vi "PolarizerRotator.vi"() -> ()   [LabVIEW 2022 SP3]
uses:
  Control_rotator.ctl
  <vilib>/Analysis/baseanly.llb/Mean (DBL).vi
  <vilib>/Analysis/NI_AALBase.lvlib
panel:
  out "error out":errorcluster
  out "concatenated string":string="0mr000007C6"
  out "Waveform Graph 2":dbl[](graph)=[0.0114104102289922, 0.005331864005048672, 0.002365437653122095, 0.0020399943555791337, 0.0018238947466399568, 0.0038770713125236265, 0.009183223773610314, 0.017346081821373458, 0.028008969359547123, 0.040766102580344826, 0.056787694052, 0.07599250286066472, 0.09984112907767431, 0.12767396257315167, 0.15908169019639953, 0.1934532823915446, 0.22536977633845853, 0.25900355543902787, 0.2854221431566561, 0.31011831747145174, 0.3226821647724511, 0.32980024781774636, 0.3281776128886943, 0.3166476606516057, 0.2977695101545653, 0.26886629570979925, 0.24020462092063113, 0.20869158381742006, 0.1768178373750466, 0.146450811441169, 0.11622057138066992, 0.09032385739868065, 0.06709021181202998, 0.04842705992607135, 0.03356983053430435, 0.021401558819280752, 0.012115542962350739]
  out "Waveform Graph":dbl[](graph)
  in  "Divide":bool
  in  "Store reference":bool
  out "String":string="000007C6"
  in  "Jog size (degrees)":dbl=5.0
  in  "Set jog size":bool
  in  "Cancel":bool
  in  "Sweep angle":dbl=180.0
  out "Current angle":i32=180
  in  "Home":bool
  in  "stop":bool
  in  "Jog":bool
  in  "milliseconds to wait":u32=1000
  out "read buffer":string="0POFFFFFFFD\r\n"
  in  "VISA resource name":refnum<visa-resource-name>="COM3"
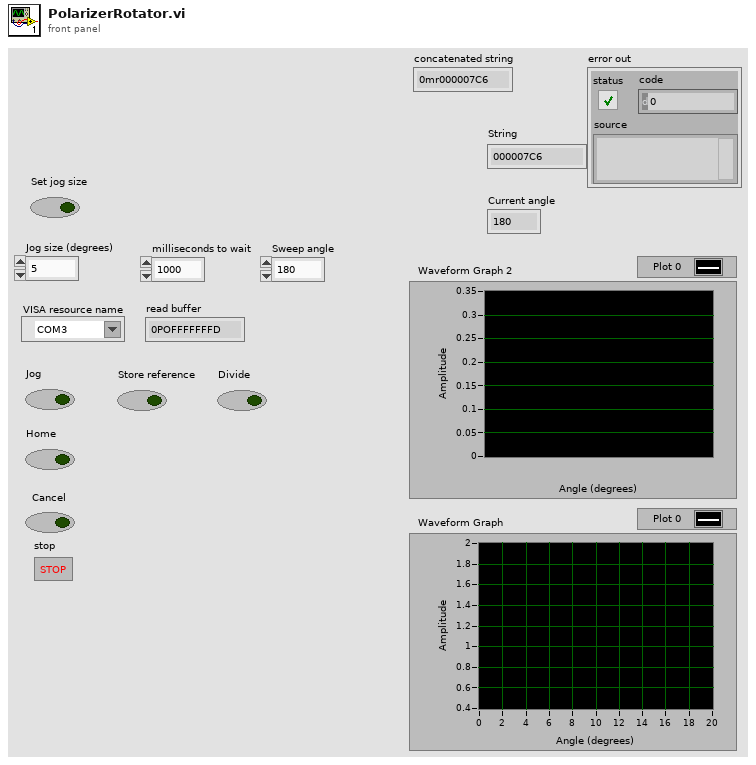
[diagram p1: front panel]
types:
  T1 = typedef "Control_rotator.ctl" = enum16{"Sit Idle", "Jog", "Set Jog Size", "Home", "Store reference", "Divide"}
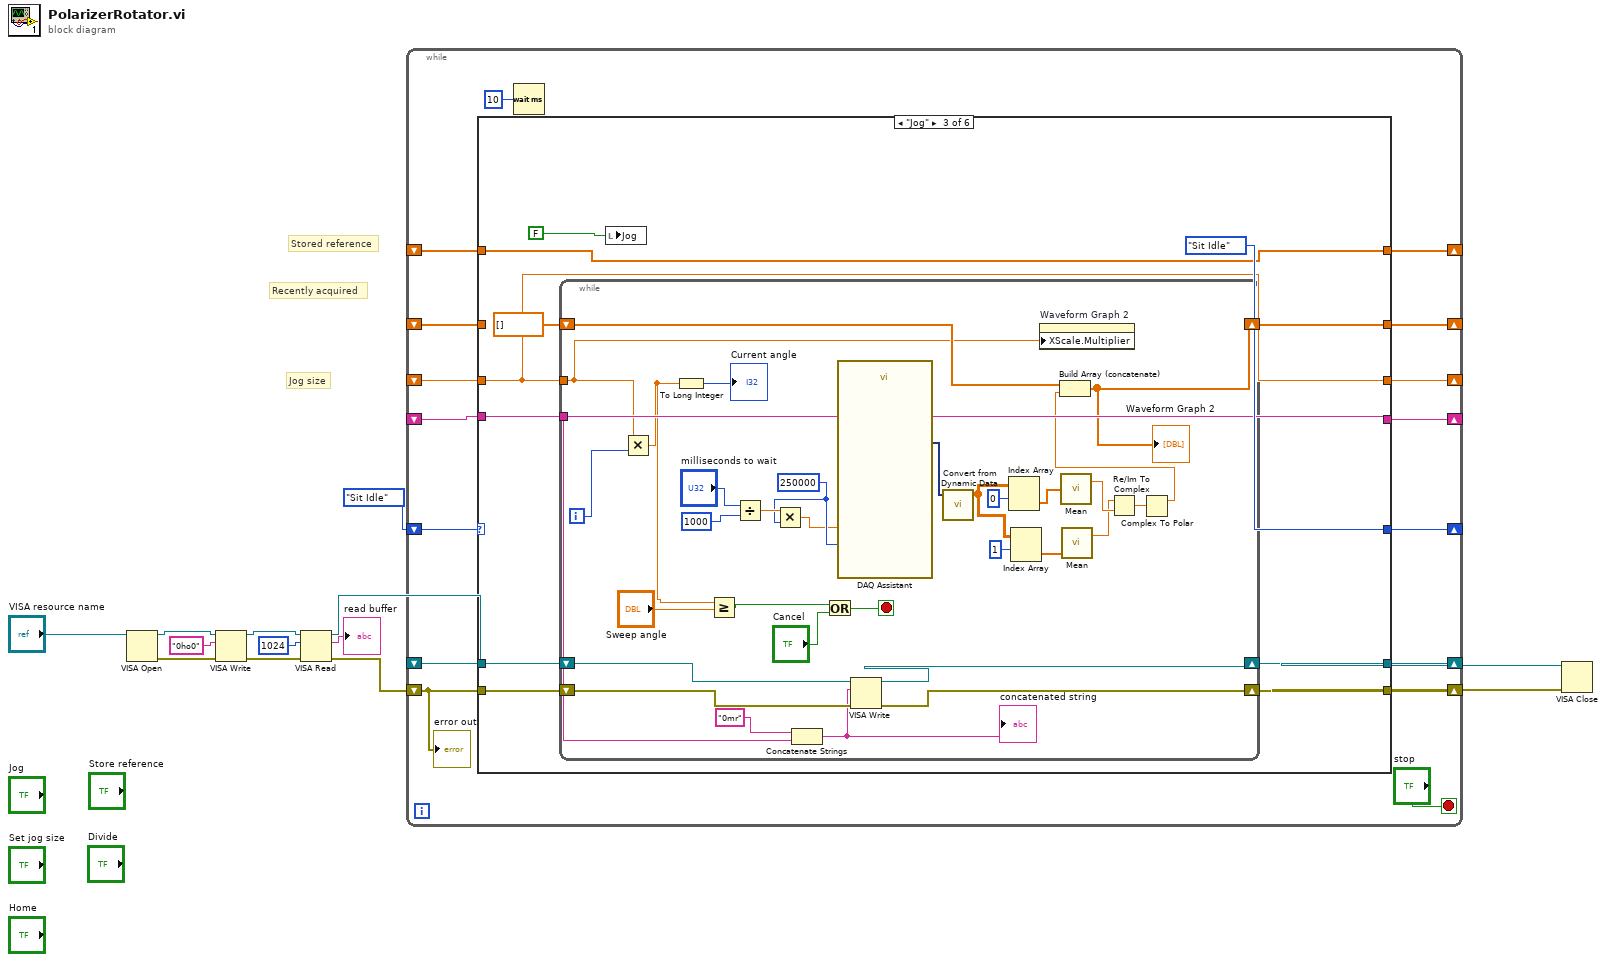
[diagram p0: block diagram]
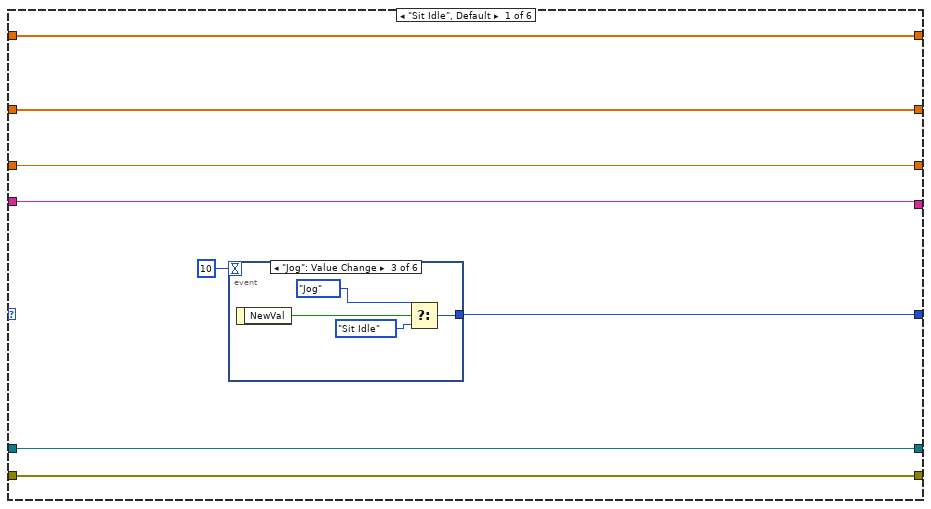
[diagram p2: hidden frame]
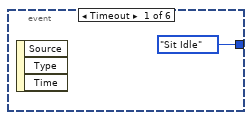
[diagram p3: hidden frame]
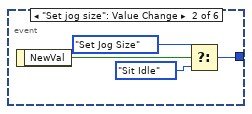
[diagram p4: hidden frame]
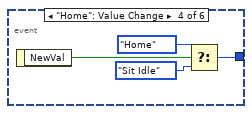
[diagram p5: hidden frame]
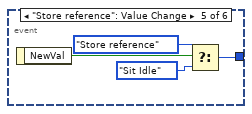
[diagram p6: hidden frame]
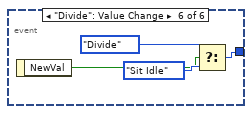
[diagram p7: hidden frame]
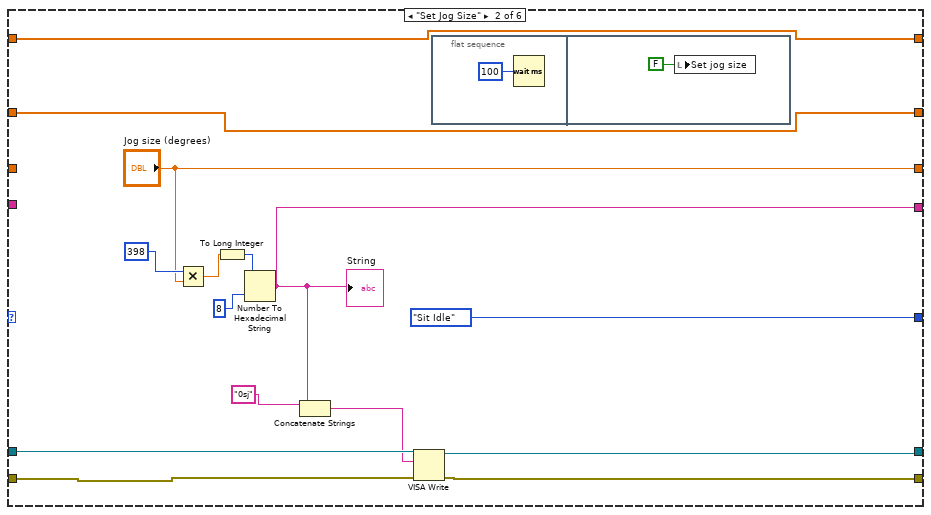
[diagram p8: hidden frame]
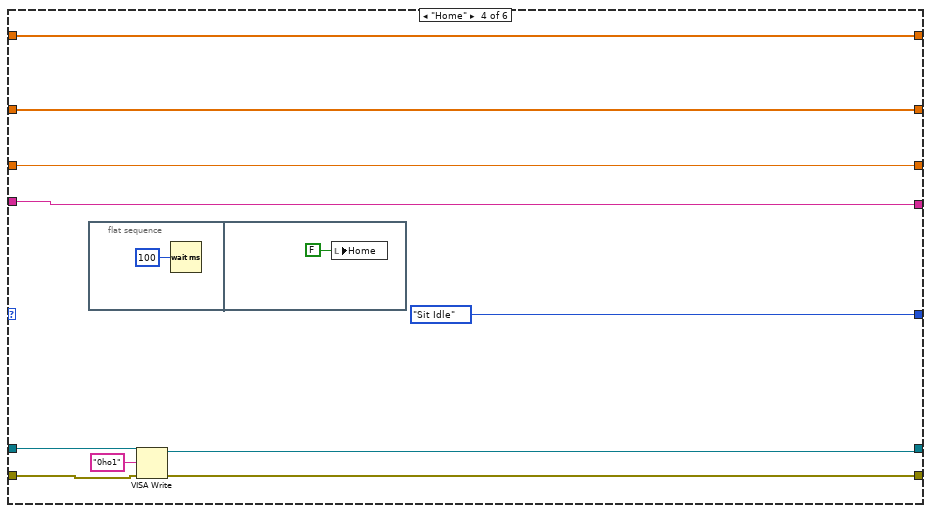
[diagram p9: hidden frame]
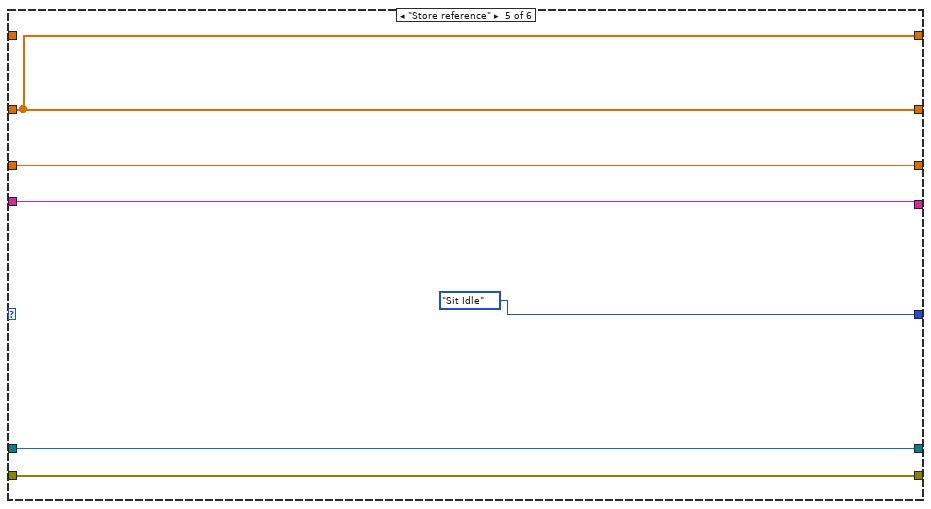
[diagram p10: hidden frame]
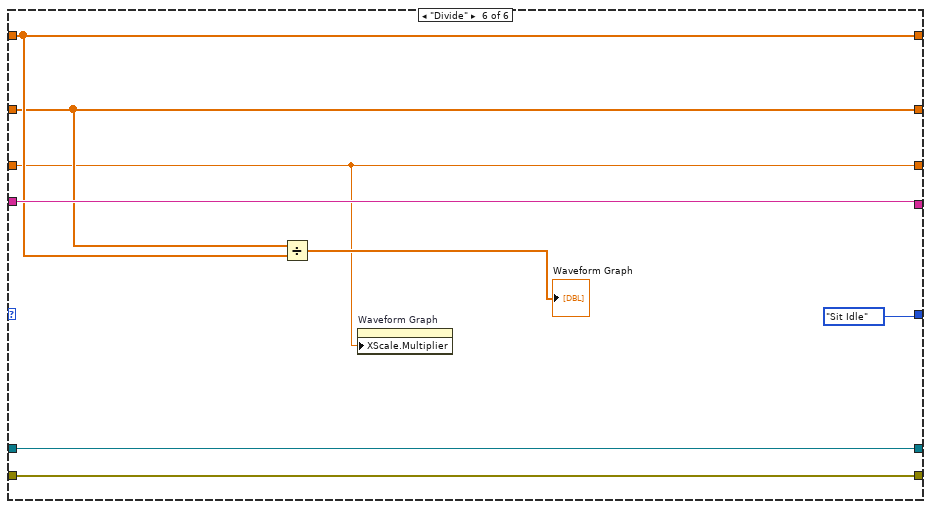
[diagram p11: hidden frame]
diagram:
  # "Jog size"
  # "Recently acquired"
  # "Stored reference"
  n1 = VISA Open(VISA resource name="VISA resource name") -> (VISA resource name=w12:refnum<visa-resource-name>, error out=w11:errorcluster)  [unwired: 4 in]
  n2 = VISA Write(VISA resource name=w12, write buffer="0ho0", error in (no error)=w11) -> (VISA resource name out=w9:refnum<visa-resource-name>, error out=w6:errorcluster)  [unwired: 1 out]
  n3 = VISA Read(VISA resource name=w9, byte count=u32 1024, error in (no error)=w6) -> (VISA resource name out=w5:refnum<visa-resource-name>, read buffer=→"read buffer":string, error out=w3:errorcluster)  [unwired: 1 out]
  n4 = while {
    shift-right: [w28] -> w4
    shift-left: w5 -> [w29]
    shift-right: [w27] -> w2
    shift-left: w3 -> [w14]
    shift-right: [w25] -> _
    shift-left: Control_rotator."Sit Idle" -> [w26]
    shift-right: [w22] -> _
    shift-left: _ -> [w23]
    shift-right: [w21] -> _
    shift-left: _ -> [w20]
    shift-right: [w18] -> _
    shift-left: _ -> [w17]
    shift-right: [w16] -> _
    shift-left: _ -> [w15]
    stop <- "stop" stop-if-true
    n5 = case shown="\"Jog\"" w26 {
      tunnel: w29 -> [w36 w73 w82 w127 w135 w143]
      tunnel: [w36 w71 w86 w124 w135 w143] -> w28
      tunnel: w14 -> [w35 w72 w81 w126 w134 w142]
      tunnel: [w35 w70 w85 w125 w134 w142] -> w27
      tunnel: [w37 Control_rotator."Sit Idle" Control_rotator."Sit Idle" Control_rotator."Sit Idle" Control_rotator."Sit Idle" Control_rotator."Sit Idle"] -> w25
      tunnel: w23 -> [w33 _ w80 w122 w133 w144]
      tunnel: [w33 w61 w80 w122 w133 w144] -> w22
      tunnel: [w32 "Jog size (degrees)" w79 w121 w132 w137] -> w21
      tunnel: w20 -> [w32 _ w79 w121 w132 w137]
      tunnel: [w31 w60 w77 w120 w131 w139] -> w18
      tunnel: w17 -> [w31 w60 _ w120 w131 w139]
      tunnel: [w30 w59 w76 w119 w131 w140] -> w16
      tunnel: w15 -> [w30 w59 w76 w119 _ w140]
      frame "Sit Idle", Default {
        n6 = event shown="[2] \"Jog\": Value Change" {
          selector: _ -> [_ _ _ _ _ _]
          dyn-events: _ -> [_ _ _ _ _ _]
          timeout: u32 10 ("milliseconds to wait") -> [_ _ _ _ _ _]
          tunnel: [Control_rotator."Sit Idle" w40 w44 w47 w52 w55] -> w37
          event Timeout {
            n7 = event-data() -> ()  [unwired: 1 in, 3 out]
          }
          event "Set jog size": Value Change {
            n8 = event-data() -> ("NewVal"=w41:bool)  [unwired: 1 in]
            n9 = Select(t=Control_rotator."Set Jog Size", s=w41, f=Control_rotator."Sit Idle") -> (s? t:f=w40:T1)
          }
          event "Jog": Value Change {
            n10 = event-data() -> ("NewVal"=w46:bool)  [unwired: 1 in]
            n11 = Select(t=Control_rotator."Jog", s=w46, f=Control_rotator."Sit Idle") -> (s? t:f=w44:T1)
          }
          event "Home": Value Change {
            n12 = event-data() -> ("NewVal"=w50:bool)  [unwired: 1 in]
            n13 = Select(t=Control_rotator."Home", s=w50, f=Control_rotator."Sit Idle") -> (s? t:f=w47:T1)
          }
          event "Store reference": Value Change {
            n14 = event-data() -> ("NewVal"=w51:bool)  [unwired: 1 in]
            n15 = Select(t=Control_rotator."Store reference", s=w51, f=Control_rotator."Sit Idle") -> (s? t:f=w52:T1)
          }
          event "Divide": Value Change {
            n16 = event-data() -> ("NewVal"=w56:bool)  [unwired: 1 in]
            n17 = Select(t=Control_rotator."Divide", s=w56, f=Control_rotator."Sit Idle") -> (s? t:f=w55:T1)
          }
        }
      }
      frame "Set Jog Size" {
        n18 = Multiply(x=398, y="Jog size (degrees)") -> (x*y=w65:dbl)
        n19 = To Long Integer(number=w65) -> (32bit integer=w66:i32)
        n20 = Number To Hexadecimal String(1:i16 8 ("width (-)"), 2:w66) -> (0:w61:string)
        "String" <- w61
        n21 = Concatenate Strings("0sj" ("string"), w61) -> (w67:string)
        n22 = VISA Write(VISA resource name=w73, write buffer=w67, error in (no error)=w72) -> (VISA resource name out=w71:refnum<visa-resource-name>, error out=w70:errorcluster)  [unwired: 1 out]
        n23 = flat-sequence {
          frame #0 {
            n24 = Wait (ms)(milliseconds to wait=u32 100) -> ()  [unwired: 1 out]
          }
          frame #1 {
            n25 = local write "Set jog size"(FALSE) -> ()
          }
        }
      }
      frame "Jog" {
        n26 = while {
          shift-right: [w118] -> w86
          shift-left: w82 -> [w116]
          shift-right: [w117] -> w85
          shift-left: w81 -> [w115]
          tunnel: w80 -> [w111]
          tunnel: w79 -> [w103]
          shift-right: [w104] -> w77
          shift-left: dbl[] [] ("History Data") -> [w106]
          i -> [w105]
          stop <- w114 stop-if-true
          w97 = 250000
          n27 = Multiply(x=w103, y=w105) -> (x*y=w107:dbl)
          n28 = To Long Integer(number=w107) -> (32bit integer=→"Current angle":i32)
          n29 = Greater Or Equal?(x=w107, y="Sweep angle") -> (x >= y?=w109:bool)
          n30 = Divide(x="milliseconds to wait", y=u32 1000) -> (x/y=w98:dbl)
          n31 = Multiply(x=w98, y=w97) -> (x*y=w96:dbl)
          n32 = Concatenate Strings("0mr" ("write buffer"), w111) -> (w102:string)
          "concatenated string" <- w102
          n33 = Or(x=w109, y="Cancel") -> (x .or. y?=w114:bool)
          n34 = call "DAQ Assistant"("rate"=w97, "number of samples"=w96) -> ("data"=w101:dynamicdata)  [unwired: 15 in, 2 out]
          n35 = VISA Write(VISA resource name=w116, write buffer=w102, error in (no error)=w115) -> (VISA resource name out=w118:refnum<visa-resource-name>, error out=w117:errorcluster)  [unwired: 1 out]
          n36 = call "Convert from Dynamic Data"("Dynamic Data Type"=w101) -> ("Array"=w93:dbl[][])  [unwired: 3 in]
          n37 = Index Array(array=w93, index (row)=0) -> (element=w92:dbl[])  [unwired: 1 in]
          n38 = Index Array(array=w93, index (row)=1) -> (element=w91:dbl[])  [unwired: 1 in]
          n39 = property on="Waveform Graph 2" class="WFGraph (strict)"("XScale.Multiplier"=w103) -> ()  [unwired: 2 in, 2 out]
          n40 = call-poly <vilib>:"Mean.vi"("X"=w92) -> ("mean"=w90:dbl)  [unwired: 1 out]
          n41 = call-poly <vilib>:"Mean.vi"("X"=w91) -> ("mean"=w89:dbl)  [unwired: 1 out]
          n42 = Re/Im To Complex(1:w90, 2:w89) -> (0:w88:cdb)
          n43 = Complex To Polar(r * e^(i*theta)=w88) -> (r=w87:dbl)  [unwired: 1 out]
          n44 = Build Array (concatenate)(w106, w87) -> (w104:dbl[])
          "Waveform Graph 2" <- w104
        }
        n45 = local write "Jog"(FALSE ("Run Scan")) -> ()
      }
      frame "Home" {
        n46 = flat-sequence {
          frame #0 {
            n47 = Wait (ms)(milliseconds to wait=u32 100) -> ()  [unwired: 1 out]
          }
          frame #1 {
            n48 = local write "Home"(FALSE ("Home")) -> ()
          }
        }
        n49 = VISA Write(VISA resource name=w127, write buffer="0ho1", error in (no error)=w126) -> (VISA resource name out=w124:refnum<visa-resource-name>, error out=w125:errorcluster)  [unwired: 1 out]
      }
      frame "Store reference" {
      }
      frame "Divide" {
        n50 = Divide(x=w139, y=w140) -> (x/y=→"Waveform Graph":dbl[])
        n51 = property on="Waveform Graph" class="WFGraph (strict)"("XScale.Multiplier"=w137) -> ()  [unwired: 2 in, 2 out]
      }
    }
    n52 = Wait (ms)(milliseconds to wait=u32 10) -> ()  [unwired: 1 out]
    "error out" <- w14
  }
  n53 = VISA Close(VISA resource name=w4, error in (no error)=w2) -> ()  [unwired: 1 out]
